vi "GetText.vi"(8 "error in (no error)":errorcluster, 11 "Text in":refnum<class "Text.lvclass">) -> (0 "error out":errorcluster, 2 "Text":string, 3 "Text out":refnum<class "Text.lvclass">)   [LabVIEW 2021, in "Picture2D.lvlib" / "Text.lvclass"]
uses:
  Text.lvclass
  Text.lvclass/Text.ctl
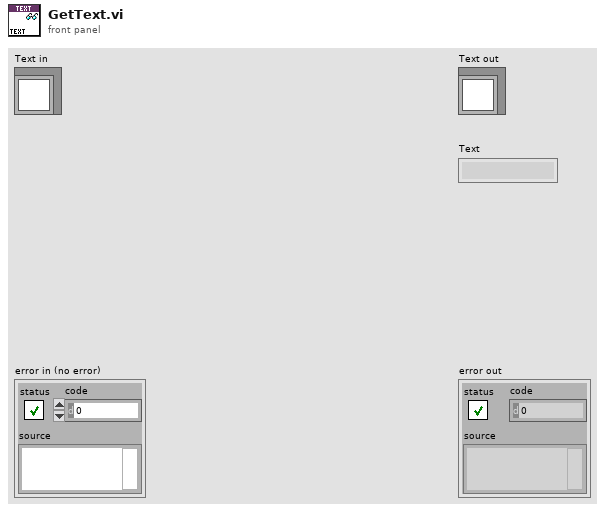
[diagram p1: front panel]
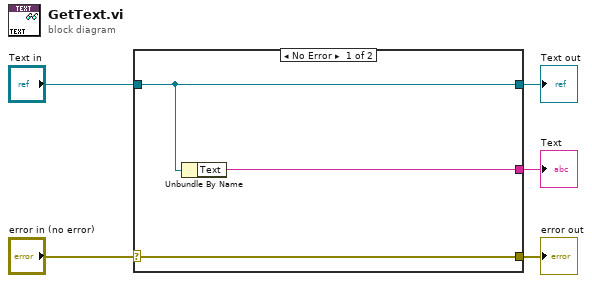
[diagram p0: block diagram]
diagram:
  n1 = case shown="No Error" "error in (no error)" {
    selector: "error in (no error)" -> [w8 w9]
    tunnel: [w8 w9] -> w4
    tunnel: [w7 w10] -> w2
    tunnel: "Text in" -> [w7 w10]
    tunnel: [w6 _] -> w1
    frame No Error {
      n2 = Unbundle By Name(w7) -> ("Text"=w6:string)
    }
    frame Error {
    }
  }
  "error out" <- w4
  "Text out" <- w2
  "Text" <- w1
